vi "manual_random.vi"(5 "change_in_event":refnum<user-event>, 7 "transition_queue":refnum<queue>, 8 "error in (no error)":errorcluster, 11 "data":variant) -> (0 "error out":errorcluster)   [LabVIEW 2015, in "example_01.lvlib"]
uses:
  example_01.lvlib
  lv-recipe-machine/public/_controls/change.ctl
  lv-recipe-machine/public/_controls/transition.ctl
  _controls/steps_actions_data.ctl
  _controls/steps_actions.ctl
  lv-recipe-machine/lv-recipe-machine.lvlib
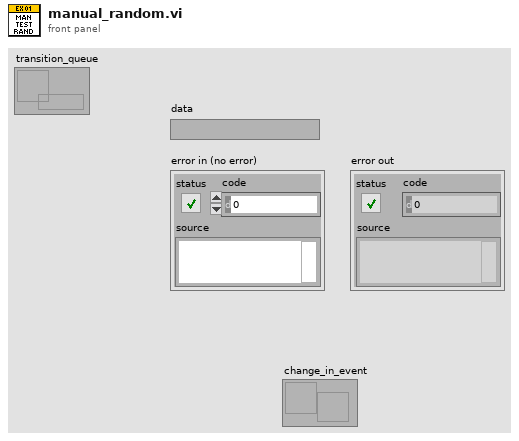
[diagram p1: front panel]
types:
  T1 = typedef "example_01.lvlib/steps_actions.ctl" = enum16{"<steps_actions>", "manual_random", "manual_comparison", "manual_wait", "auto_random", "auto_wait", "criteria_initialize", "criteria_count", "criteria_comparison", "transition_simple", "transition_count", "transition_comparison", "launch_wait", "<null>"}
  T2 = typedef "example_01.lvlib/steps_actions_data.ctl" = cluster{"step_action":T1, "data":variant}
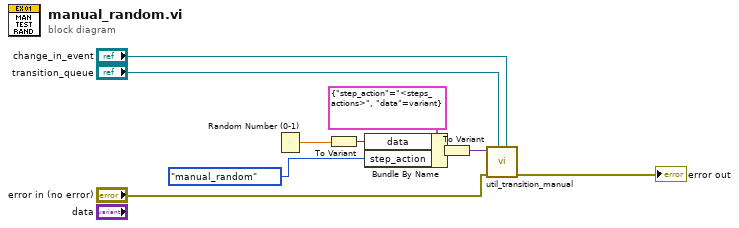
[diagram p0: block diagram]
diagram:
  n1 = Random Number (0-1)() -> (number: 0 to 1=w7:dbl)
  n2 = To Variant(anything=w7) -> (Variant=w6:variant)
  n3 = Bundle By Name(cluster=T2 {"step_action"=enum."<steps_actions>", "data"=variant}, "data"=w6, "step_action"=steps_actions."manual_random" ("manual_action")) -> (w8:T2)
  n4 = To Variant(anything=w8) -> (Variant=w5:variant)
  n5 = call "util_transition_manual.vi"("change_in_event"="change_in_event", "transition_queue"="transition_queue", "error in (no error)"="error in (no error)", "data"=w5) -> ("error out"=→"error out":errorcluster)  [unwired: 7 in]
